vi "Exercise 6_13.vi"() -> ()   [LabVIEW 2018]
uses:
  <vilib>/Utility/file.llb/Read Delimited Spreadsheet (DBL).vi
  <vilib>/Utility/file.llb/Write Delimited Spreadsheet (DBL).vi
panel:
  out "all rows":dbl[][](array[numeric]) caption="모든 행"
  out "웨이브폼 차트":dbl[][](graph)
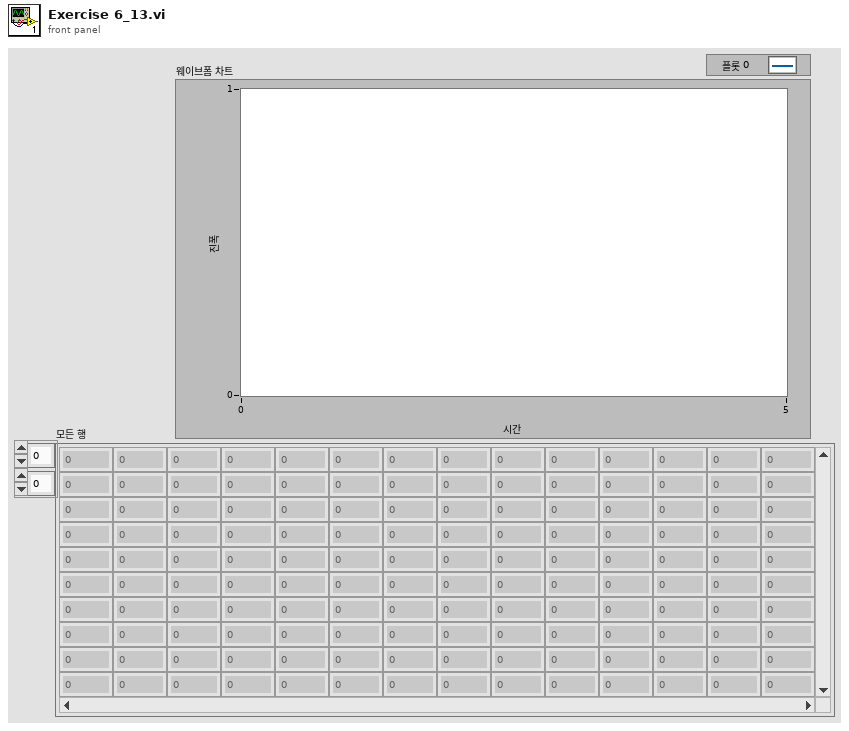
[diagram p1: front panel]
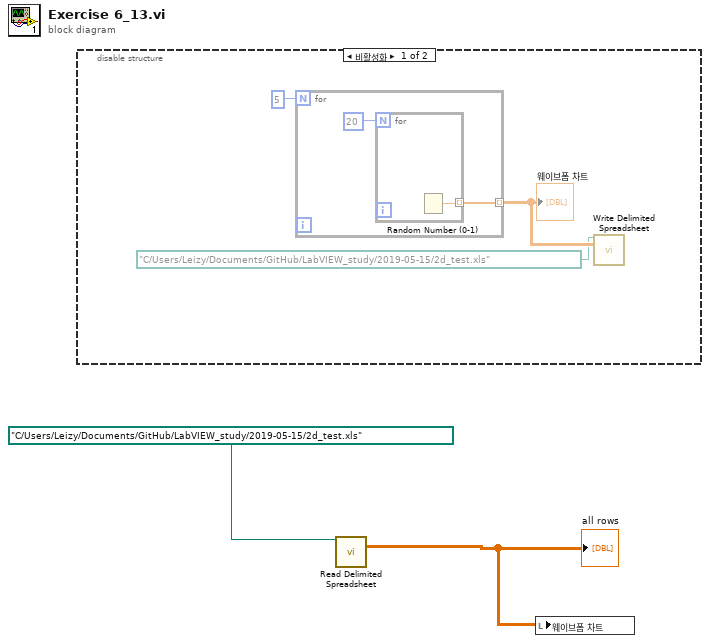
[diagram p0: block diagram]
diagram:
  n1 = disable-structure shown="비활성화" {
    frame Disabled {
      n2 = for {
        N: 5 -> [_]
        tunnel: [w6] -> w4 mode=indexing
        n3 = for {
          N: 20 -> [_]
          tunnel: [w8] -> w6 mode=indexing
          n4 = Random Number (0-1)() -> (number: 0 to 1=w8:dbl)
        }
      }
      "웨이브폼 차트" <- w4
      n5 = call-poly <vilib>:"Write Delimited Spreadsheet.vi"("file path (dialog if empty)"=path "C:/Users/Leizy/Documents/GitHub/LabVIEW_study/2019-05-15/2d_test.xls", "2D data"=w4) -> ()  [unwired: 12 in, 2 out]
    }
    frame Enabled {
    }
  }
  n6 = call-poly <vilib>:"Read Delimited Spreadsheet.vi"("file path (dialog if empty)"=path "C:/Users/Leizy/Documents/GitHub/LabVIEW_study/2019-05-15/2d_test.xls") -> ("all rows"=w1:dbl[][])  [unwired: 9 in, 5 out]
  "all rows" <- w1
  n7 = local write "웨이브폼 차트"(w1) -> ()
